vi "BinaryRectangleDetector.vi"(0 "Image In":T2, 7 "error in":errorcluster) -> (20 "Image Out":T2, 21 "distance":dbl, 22 "theta":dbl, 23 "deltax":dbl, 24 "deltay":dbl, 27 "error out":errorcluster)   [LabVIEW 2011]
uses:
  <vilib>/vision/Image Controls.llb/IMAQ Image.ctl
  <vilib>/vision/Measure.llb/Edge Options.ctl
  <vilib>/vision/Measure.llb/Edge Polarity.ctl
  <vilib>/vision/Measure.llb/Straight Edge Options.ctl
  <vilib>/vision/Measure.llb/Straight Edge Process.ctl
  <vilib>/vision/NI_Vision_Development_Module.lvlib
  <vilib>/Analysis/NI_AALBase.lvlib
panel:
  in  "Use Simple":bool
  out "Simple Height":dbl
  out "Simple Width":dbl
  in  "db":dbl=3.0
  in  "thresh":dbl=300.0
  out "width":sgl
  out "height":sgl
  in  "d0":dbl=115.0
  in  "p0":dbl=63.0
  in  "Rectangle":T1 {"Rotation" format="%.2f"; "Left" scale=0.0..1024.0; "Right" scale=0.0..1024.0}
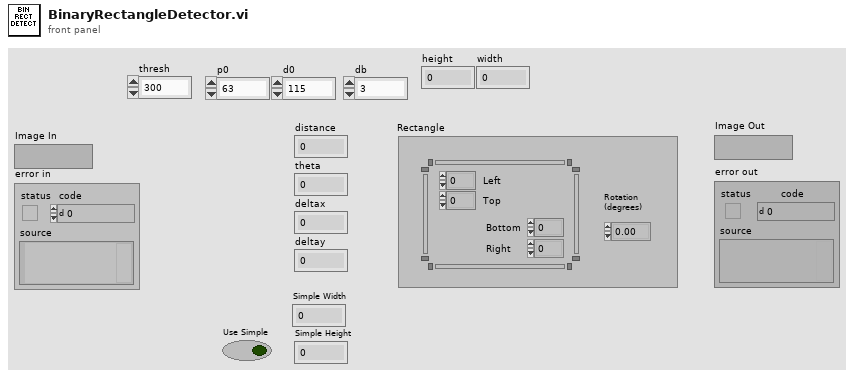
[diagram p1: front panel]
types:
  T1 = typedef "IMAQ Rectangle" = cluster{"Left":i32, "Top":i32, "Right":i32, "Bottom":i32, "Rotation":dbl}
  T2 = typedef "IMAQ Image.ctl" = refnum<image>
  T3 = cluster{"Feature":u32, "Points IDs":cluster{"GUID":string, "Index":i32}[]}[]
  T4 = typedef "Edge Options.ctl" = cluster{"Edge Polarity":T5, "Kernel Size":u32, "Width":u32, "Minimum Edge Strength":sgl, "Interpolation Type":enum32{"Zero Order", "Bilinear", "Quadratic", "Cubic", "Bilinear Fixed"}, "Data Processing Method":enum32{"Average", "Median"}}
  T5 = typedef "Edge Polarity.ctl" = u32
  T6 = cluster{"Search Direction":u32, "Edge Options":T4, "Show Search Area":bool, "Show Search Lines":bool, "Show Edges Found":bool, "Show Result":bool, "Search Area Color":u32, "Search Lines Color":u32, "Edge Locations Color":u32, "Result Color":u32, "Overlay Group Name":string}
  T7 = typedef "Straight Edge Options.ctl" = cluster{"Number of Lines":i32, "Type":T8, "Min. Score":dbl, "Max. Score":dbl, "Orientation":dbl, "Angle Range":dbl, "Angle Tolerance":dbl, "Step Size":u32, "Min. SNR (db)":dbl, "Min. Points (%)":dbl, "Hough Iterations":i32}
  T8 = typedef "Straight Edge Process.ctl" = enum32{"First Edge Rake", "Best Edge Rake", "Hough Edge Rake", "First Edge Projection", "Best Edge Projection"}
  T9 = typedef "ROI Descriptor" = cluster{"Global Rectangle":i32[], "Contours":cluster{"ID":enum32{"External", "Internal"}, "Type":u32, "Coordinates":i32[]}[]}
  T10 = cluster{"histogram":u32[], "Minimal Value":sgl, "Maximal Value":sgl, "Starting Value":sgl, "Interval Width":sgl, "Mean Value":sgl, "Standard  Variation":sgl, "Area (pixels)":i32}
  T11 = typedef "Image Type" = u32
  T12 = cluster{"Point1 (Pixels)":cluster{"X":sgl, "Y":sgl}, "Point2 (Pixels)":cluster{"X":sgl, "Y":sgl}, "Point1 (Real-World)":cluster{"X":sgl, "Y":sgl}, "Point2 (Real-World)":cluster{"X":sgl, "Y":sgl}, "Angle (Pixel)":dbl, "Angle (Real-World)":dbl, "Score":dbl, "Straightness":dbl, "Average SNR (db)":dbl, "Calibration Valid":bool}[]
  T13 = cluster{"Point1 (Pixels)":cluster{"X":sgl, "Y":sgl}, "Point2 (Pixels)":cluster{"X":sgl, "Y":sgl}, "Point1 (Real-World)":cluster{"X":sgl, "Y":sgl}, "Point2 (Real-World)":cluster{"X":sgl, "Y":sgl}, "Angle (Pixel)":dbl, "Angle (Real-World)":dbl, "Score":dbl, "Straightness":dbl, "Average SNR (db)":dbl, "Calibration Valid":bool}
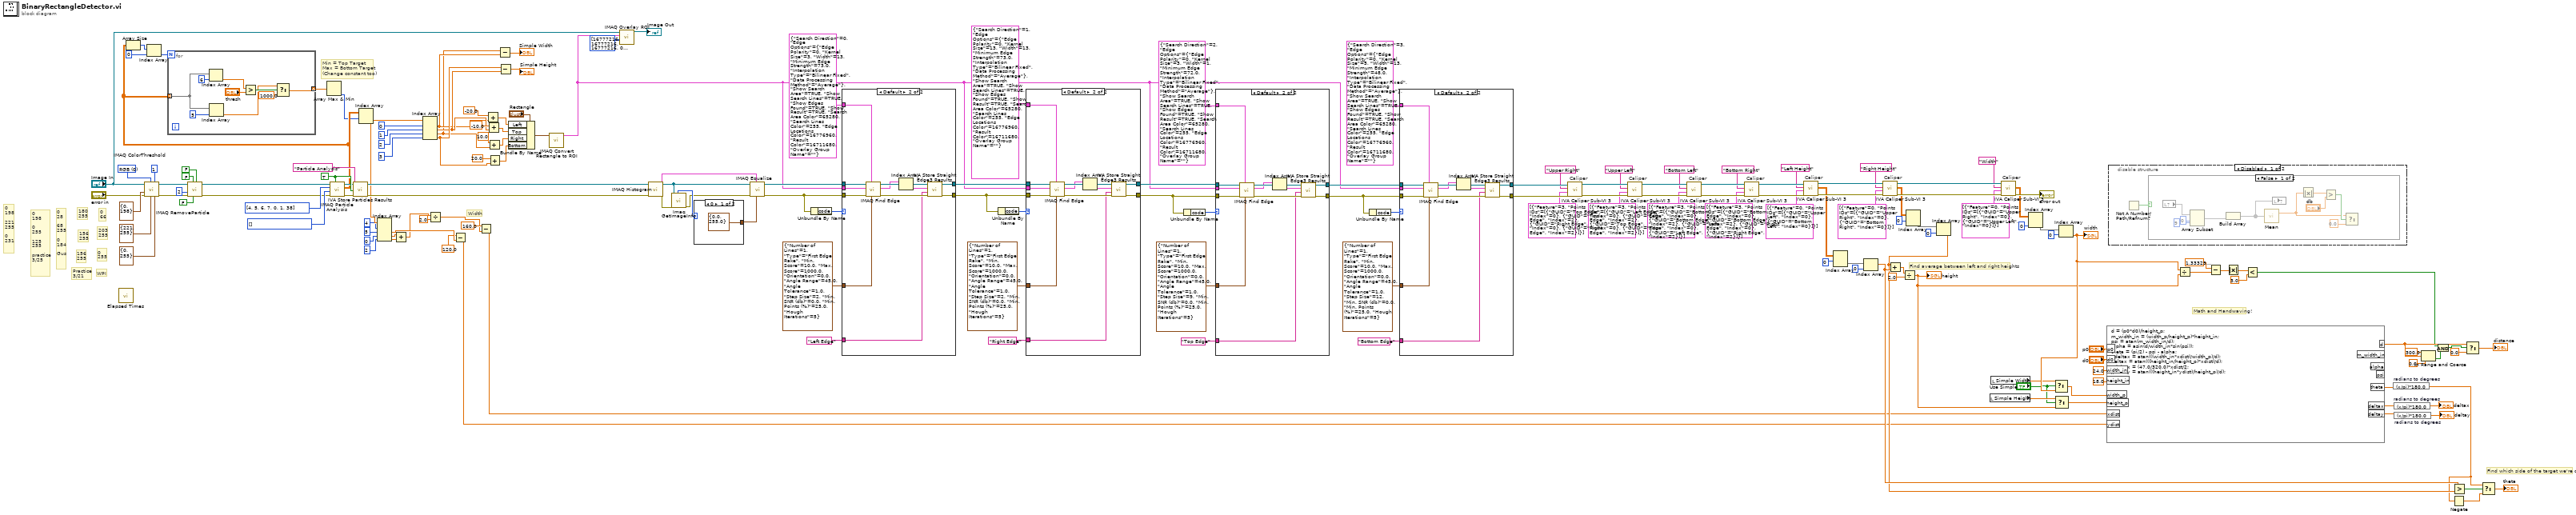
[diagram p0: block diagram]
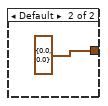
[diagram p8: hidden frame]
diagram:
  w162 = i32[] [] items=["Center of Mass X", "Center of Mass Y", "First Pixel X", "First Pixel Y", "Bounding Rect Left", "Bounding Rect Top", "Bounding Rect Right", "Bounding Rect Bottom", "Max Feret Diameter Start X", "Max Feret Diameter Start Y", "Max Feret Diameter End X", "Max Feret Diameter End Y", "Max Horiz. Segment Length Left", "Max Horiz. Segment Length Right", "Max Horiz. Segment Length Row", "-", "Bounding Rect Width", "Bounding Rect Height", "Bounding Rect Diagonal", "Perimeter", "Convex Hull Perimeter", "Holes' Perimeter", "Max Feret Diameter", "Equivalent Ellipse Major Axis", "Equivalent Ellipse Minor Axis", "Equivalent Ellipse Minor Axis (Feret)", "Equivalent Rect Long Side", "Equivalent Rect Short Side", "Equivalent Rect Diagonal", "Equivalent Rect Short Side (Feret)", "Average Horiz. Segment Length", "Average Vert. Segment Length", "Hydraulic Radius", "Waddel Disk Diameter", "-", "Area", "Holes' Area", "Particle & Holes' Area", "Convex Hull Area", "Image Area", "-", "Number of Holes", "Number of Horiz. Segments", "Number of Vert. Segments", "-", "Orientation", "Max Feret Diameter Orientation", "-", "% Area/Image Area", "% Area/(Particle & Holes' Area)", "Ratio of Equivalent Ellipse Axes", "Ratio of Equivalent Rect Sides", "-", "Elongation Factor", "Compactness Factor", "Heywood Circularity Factor", "Type Factor", "-", "Sum X", "Sum Y", "Sum XX", "Sum XY", "Sum YY", "Sum XXX", "Sum XXY", "Sum XYY", "Sum YYY", "-", "Moment of Inertia XX", "Moment of Inertia XY", "Moment of Inertia YY", "Moment of Inertia XXX", "Moment of Inertia XXY", "Moment of Inertia XYY", "Moment of Inertia YYY", "Norm. Moment of Inertia XX", "Norm. Moment of Inertia XY", "Norm. Moment of Inertia YY", "Norm. Moment of Inertia XXX", "Norm. Moment of Inertia XXY", "Norm. Moment of Inertia XYY", "Norm. Moment of Inertia YYY", "Hu Moment 1", "Hu Moment 2", "Hu Moment 3", "Hu Moment 4", "Hu Moment 5", "Hu Moment 6", "Hu Moment 7"] ("Real-World Measurements")
  w163 = i32[] [4, 5, 6, 7, 0, 1, 38] items=["Center of Mass X", "Center of Mass Y", "First Pixel X", "First Pixel Y", "Bounding Rect Left", "Bounding Rect Top", "Bounding Rect Right", "Bounding Rect Bottom", "Max Feret Diameter Start X", "Max Feret Diameter Start Y", "Max Feret Diameter End X", "Max Feret Diameter End Y", "Max Horiz. Segment Length Left", "Max Horiz. Segment Length Right", "Max Horiz. Segment Length Row", "-", "Bounding Rect Width", "Bounding Rect Height", "Bounding Rect Diagonal", "Perimeter", "Convex Hull Perimeter", "Holes' Perimeter", "Max Feret Diameter", "Equivalent Ellipse Major Axis", "Equivalent Ellipse Minor Axis", "Equivalent Ellipse Minor Axis (Feret)", "Equivalent Rect Long Side", "Equivalent Rect Short Side", "Equivalent Rect Diagonal", "Equivalent Rect Short Side (Feret)", "Average Horiz. Segment Length", "Average Vert. Segment Length", "Hydraulic Radius", "Waddel Disk Diameter", "-", "Area", "Holes' Area", "Particle & Holes' Area", "Convex Hull Area", "Image Area", "-", "Number of Holes", "Number of Horiz. Segments", "Number of Vert. Segments", "-", "Orientation", "Max Feret Diameter Orientation", "-", "% Area/Image Area", "% Area/(Particle & Holes' Area)", "Ratio of Equivalent Ellipse Axes", "Ratio of Equivalent Rect Sides", "-", "Elongation Factor", "Compactness Factor", "Heywood Circularity Factor", "Type Factor", "-", "Sum X", "Sum Y", "Sum XX", "Sum XY", "Sum YY", "Sum XXX", "Sum XXY", "Sum XYY", "Sum YYY", "-", "Moment of Inertia XX", "Moment of Inertia XY", "Moment of Inertia YY", "Moment of Inertia XXX", "Moment of Inertia XXY", "Moment of Inertia XYY", "Moment of Inertia YYY", "Norm. Moment of Inertia XX", "Norm. Moment of Inertia XY", "Norm. Moment of Inertia YY", "Norm. Moment of Inertia XXX", "Norm. Moment of Inertia XXY", "Norm. Moment of Inertia XYY", "Norm. Moment of Inertia YYY", "Hu Moment 1", "Hu Moment 2", "Hu Moment 3", "Hu Moment 4", "Hu Moment 5", "Hu Moment 6", "Hu Moment 7"] ("Pixel Measurements")
  w161 = TRUE ("Connectivity 4/8 (8)")
  w173 = u16 0 items=["RGB", "HSL", "HSV", "HSI"] ("Color Mode")
  # "Width"
  # "0\n198\n\n221\n255\n\n0\n231"
  # "0\n198\n\n0\n255\n\n125\n255\n\npractice\n3/25"
  # "0\n28\n\n68\n255\n\n0\n184\n\nGus"
  # "Practice\n3/21"
  # "WPI"
  # "156\n255"
  # "156\n255"
  # "180\n255"
  # "0\n255"
  # "203\n255"
  # "0\n66"
  # "Min = Top Target\nMax = Bottom Target\n(Change constant too)"
  # "Find average between left and right heights"
  # "Math and Handwaving!"
  # "Find which side of the target we're on"
  # "Caliper"
  # "Caliper"
  # "Caliper"
  # "Caliper"
  # "Caliper"
  # "Caliper"
  # "Caliper"
  n1 = call "Elapsed Times.vi"() -> ()  [unwired: 3 in, 1 out]
  n2 = call "IMAQ ColorThreshold"("Blue or Luma or Val or Inten Range"=cluster{"Lower value":i32, "Upper value":i32} {"Lower value"=0, "Upper value"=255}, "Replace Value"=1, "Green or Sat Range"=cluster{"Lower value":i32, "Upper value":i32} {"Lower value"=221, "Upper value"=255}, "Color Mode"=w173, "error in (no error)"="error in", "Red or Hue Range"=cluster{"Lower value":i32, "Upper value":i32} {"Lower value"=0, "Upper value"=198}, "Image Src"="Image In") -> ("error out"=w168:errorcluster, "Image Dst Out"=w39:T2)  [unwired: 1 in, 2 out]
  n3 = call "IMAQ RemoveParticle"("Connectivity 4/8 (8)"=FALSE, "Low Pass/High Pass (Low)"=FALSE, "Square/Hexa (Square)"=FALSE, "error in (no error)"=w168, "Number of Erosion"=2, "Image Src"=w39) -> ("error out"=w41:errorcluster, "Image Dst Out"=w42:T2)  [unwired: 1 in, 3 out]
  n4 = call "IMAQ Particle Analysis"("Connectivity 4/8 (8)"=w161, "error in (no error)"=w41, "Real-World Measurements"=w162, "Pixel Measurements"=w163, "Image"=w42) -> ("error out"=w158:errorcluster, "Particle Measurements (Pixels)"=w36:dbl[][], "Image Out (duplicate)"=w160:T2)  [unwired: 4 out]
  n5 = Array Size(array=w36) -> (size(s)=w50:i32[])
  n6 = Index Array(array=w50, index=0) -> (element=w48:i32)
  n7 = for {
    N: w48 -> [_]
    tunnel: w36 -> [w181] mode=indexing
    tunnel: [w175] -> w40 mode=indexing
    n8 = Index Array(array=w181, index=6) -> (element=w180:dbl)
    n9 = Index Array(array=w181, index=5) -> (element=w177:dbl)
    n10 = Greater?(x=w180, y="thresh") -> (0:w178:bool)
    n11 = Select(t=w177, s=w178, f=1000.0) -> (s? t:f=w175:dbl)
  }
  n12 = Array Max & Min(array=w40) -> (min index (indices)=w29:i32)  [unwired: 3 out]
  n13 = call <vilib>:"IVA Store Particles Results.vi"("error in (no error)"=w158, "Connectivity 4/8 (8)"=w161, "Step Name"="Particle Analysis", "Image in"=w160) -> ("error out"=w157:errorcluster, "Image dup"=w153:T2)  [unwired: 6 out]
  n14 = Index Array(array=w36, index (row)=w29) -> (element=w69:dbl[])  [unwired: 1 in]
  n15 = Index Array(array=w69, index #1=4 ("index"), index #2=5 ("index"), index #3=0 ("index"), index #4=2 ("index")) -> (element #2=w45:dbl, element #3=w5:dbl, element #4=w4:dbl)  [unwired: 1 out]
  n16 = Add(x=w5, y=w4) -> (x+y=w3:dbl)
  n17 = Index Array(array=w69, index #1=0 ("index"), index #2=1 ("index"), index #3=2 ("index"), index #4=3 ("index")) -> (element #1=w17:dbl, element #2=w18:dbl, element #3=w16:dbl, element #4=w19:dbl)
  n18 = Divide(x=w3, y=2.0) -> (x/y=w1:dbl)
  n19 = Subtract(x=120.0, y=w45) -> (x-y=w43:dbl)
  n20 = Subtract(x=160.0, y=w1) -> (x-y=w46:dbl)
  n21 = Add(x=-20.0 ("y"), y=w17) -> (x+y=w90:dbl)
  n22 = Add(x=-10.0, y=w18) -> (x+y=w89:dbl)
  n23 = Add(x=10.0, y=w16) -> (x+y=w88:dbl)
  n24 = Add(x=20.0, y=w19) -> (x+y=w87:dbl)
  n25 = Subtract(x=w16, y=w17) -> (x-y=→"Simple Width":dbl)
  n26 = Subtract(x=w19, y=w18) -> (x-y=→"Simple Height":dbl)
  n27 = Bundle By Name(cluster="Rectangle", "Left"=w90, "Top"=w89, "Right"=w88, "Bottom"=w87) -> (w86:T1)
  n28 = call "IMAQ Convert Rectangle to ROI"("Rectangle"=w86) -> ("ROI Descriptor"=w37:T9)  [unwired: 8 in, 1 out]
  n29 = call "IMAQ Overlay ROI"("Point Symbol"=u32[][] [[16777216, 16777216, 16777216, 0, 16777216, 16777216, 16777216], [16777216, 16777216, 16777216, 0, 16777216, 16777216, 16777216], [16777216, 16777216, 16777216, 0, 16777216, 16777216, 16777216], [0, 0, 0, 16777216, 0, 0, 0], [16777216, 16777216, 16777216, 0, 16777216, 16777216, 16777216], [16777216, 16777216, 16777216, 0, 16777216, 16777216, 16777216], [16777216, 16777216, 16777216, 0, 16777216, 16777216, 16777216]], "ROI Descriptor"=w37, "Image"="Image In") -> ("Image Out"=→"Image Out":T2)  [unwired: 7 in, 1 out]
  n30 = call "IMAQ Histogram"("error in (no error)"=w157, "Image"=w153) -> ("error out"=w152:errorcluster, "Histogram Report"=w155:T10)  [unwired: 3 in, 5 out]
  n31 = call "Imaq GetImageInfo"("error in (no error)"=w152, "Image"=w153) -> ("error out"=w151:errorcluster, "Image Type"=w154:T11)  [unwired: 8 out]
  n32 = case shown="0" w154 {
    tunnel: [cluster{"Minimum":sgl, "Maximum":sgl} {"Minimum"=0.0, "Maximum"=255.0} ("Range") cluster{"Minimum":sgl, "Maximum":sgl} {"Minimum"=0.0, "Maximum"=0.0} ("Range")] -> w150
    frame 0 {
    }
    frame Default {
    }
  }
  n33 = call "IMAQ Equalize"("Range"=w150, "Histogram Report"=w155, "error in (no error)"=w151, "Image Src"=w153) -> ("error out"=w156:errorcluster, "Image Dst Out"=w85:T2)  [unwired: 2 in, 4 out]
  n34 = Unbundle By Name(w156) -> ("code"=w147:i32)
  n35 = case shown="Default" w147 {
    tunnel: w85 -> [w186 w198]
    tunnel: w156 -> [_ w197]
    tunnel: w37 -> [_ w191]
    tunnel: [w186 w195] -> w144
    tunnel: [_ w193] -> w149
    tunnel: "Left Edge" ("Step Name") -> [_ w192]
    tunnel: T7 {"Number of Lines"=1, "Type"=enum."First Edge Rake", "Min. Score"=10.0, "Max. Score"=1000.0, "Orientation"=0.0, "Angle Range"=45.0, "Angle Tolerance"=1.0, "Step Size"=2, "Min. SNR (db)"=0.0, "Min. Points (%)"=25.0, "Hough Iterations"=5} ("Fit Options") -> [_ w190]
    tunnel: T6 {"Search Direction"=0, "Edge Options"={"Edge Polarity"=0, "Kernel Size"=3, "Width"=13, "Minimum Edge Strength"=73.0, "Interpolation Type"=enum."Bilinear Fixed", "Data Processing Method"=enum."Average"}, "Show Search Area"=TRUE, "Show Search Lines"=TRUE, "Show Edges Found"=TRUE, "Show Result"=TRUE, "Search Area Color"=65280, "Search Lines Color"=255, "Edge Locations Color"=16776960, "Result Color"=16711680, "Overlay Group Name"=""} ("Options") -> [_ w189]
    frame -1074396199, -1074396198 {
      # "Discard Coordinate System Error"
    }
    frame Default {
      n36 = call "IMAQ Find Edge"("Line Fit Options"=w190, "Options"=w189, "error in (no error)"=w197, "ROI Descriptor"=w191, "Image"=w198) -> ("error out"=w194:errorcluster, "Straight Edges"=w188:T12, "Image Out"=w196:T2)  [unwired: 1 in, 3 out]
      n37 = Index Array(array=w188) -> (element=w187:T13)  [unwired: 1 in]
      n38 = call <vilib>:"IVA Store Straight Edge3 Results.vi"("error in (no error)"=w194, "Step Name"=w192, "Straight Edge"=w187, "Image in"=w196) -> ("error out"=w193:errorcluster, "Image dup"=w195:T2)  [unwired: 1 in, 5 out]
    }
  }
  n39 = Unbundle By Name(w149) -> ("code"=w141:i32)
  n40 = case shown="Default" w141 {
    tunnel: w144 -> [w199 w211]
    tunnel: w149 -> [_ w210]
    tunnel: w37 -> [_ w204]
    tunnel: [w199 w208] -> w138
    tunnel: [_ w206] -> w143
    tunnel: "Right Edge" ("Step Name") -> [_ w205]
    tunnel: T7 {"Number of Lines"=1, "Type"=enum."First Edge Rake", "Min. Score"=10.0, "Max. Score"=1000.0, "Orientation"=0.0, "Angle Range"=45.0, "Angle Tolerance"=1.0, "Step Size"=2, "Min. SNR (db)"=0.0, "Min. Points (%)"=25.0, "Hough Iterations"=5} ("Fit Options") -> [_ w203]
    tunnel: T6 {"Search Direction"=1, "Edge Options"={"Edge Polarity"=0, "Kernel Size"=13, "Width"=13, "Minimum Edge Strength"=73.0, "Interpolation Type"=enum."Bilinear Fixed", "Data Processing Method"=enum."Average"}, "Show Search Area"=TRUE, "Show Search Lines"=TRUE, "Show Edges Found"=TRUE, "Show Result"=TRUE, "Search Area Color"=65280, "Search Lines Color"=255, "Edge Locations Color"=16776960, "Result Color"=16711680, "Overlay Group Name"=""} ("Options") -> [_ w202]
    frame -1074396199, -1074396198 {
      # "Discard Coordinate System Error"
    }
    frame Default {
      n41 = call "IMAQ Find Edge"("Line Fit Options"=w203, "Options"=w202, "error in (no error)"=w210, "ROI Descriptor"=w204, "Image"=w211) -> ("error out"=w207:errorcluster, "Straight Edges"=w201:T12, "Image Out"=w209:T2)  [unwired: 1 in, 3 out]
      n42 = Index Array(array=w201) -> (element=w200:T13)  [unwired: 1 in]
      n43 = call <vilib>:"IVA Store Straight Edge3 Results.vi"("error in (no error)"=w207, "Step Name"=w205, "Straight Edge"=w200, "Image in"=w209) -> ("error out"=w206:errorcluster, "Image dup"=w208:T2)  [unwired: 1 in, 5 out]
    }
  }
  n44 = Unbundle By Name(w143) -> ("code"=w135:i32)
  n45 = case shown="Default" w135 {
    tunnel: w138 -> [w212 w224]
    tunnel: w143 -> [_ w223]
    tunnel: [w212 w221] -> w132
    tunnel: [_ w219] -> w137
    tunnel: "Top Edge" ("Step Name") -> [_ w218]
    tunnel: T7 {"Number of Lines"=1, "Type"=enum."First Edge Rake", "Min. Score"=10.0, "Max. Score"=1000.0, "Orientation"=0.0, "Angle Range"=45.0, "Angle Tolerance"=1.0, "Step Size"=9, "Min. SNR (db)"=0.0, "Min. Points (%)"=25.0, "Hough Iterations"=5} ("Fit Options") -> [_ w217]
    tunnel: T6 {"Search Direction"=2, "Edge Options"={"Edge Polarity"=0, "Kernel Size"=3, "Width"=1, "Minimum Edge Strength"=72.0, "Interpolation Type"=enum."Bilinear Fixed", "Data Processing Method"=enum."Average"}, "Show Search Area"=TRUE, "Show Search Lines"=TRUE, "Show Edges Found"=TRUE, "Show Result"=TRUE, "Search Area Color"=65280, "Search Lines Color"=255, "Edge Locations Color"=16776960, "Result Color"=16711680, "Overlay Group Name"=""} ("Options") -> [_ w216]
    tunnel: w37 -> [_ w213]
    frame -1074396199, -1074396198 {
      # "Discard Coordinate System Error"
    }
    frame Default {
      n46 = call "IMAQ Find Edge"("Line Fit Options"=w217, "Options"=w216, "error in (no error)"=w223, "ROI Descriptor"=w213, "Image"=w224) -> ("error out"=w220:errorcluster, "Straight Edges"=w215:T12, "Image Out"=w222:T2)  [unwired: 1 in, 3 out]
      n47 = Index Array(array=w215) -> (element=w214:T13)  [unwired: 1 in]
      n48 = call <vilib>:"IVA Store Straight Edge3 Results.vi"("error in (no error)"=w220, "Step Name"=w218, "Straight Edge"=w214, "Image in"=w222) -> ("error out"=w219:errorcluster, "Image dup"=w221:T2)  [unwired: 1 in, 5 out]
    }
  }
  n49 = Unbundle By Name(w137) -> ("code"=w129:i32)
  n50 = case shown="Default" w129 {
    tunnel: w132 -> [w225 w237]
    tunnel: w137 -> [_ w236]
    tunnel: w37 -> [_ w230]
    tunnel: [w225 w234] -> w126
    tunnel: [_ w232] -> w131
    tunnel: "Bottom Edge" ("Step Name") -> [_ w231]
    tunnel: T7 {"Number of Lines"=1, "Type"=enum."First Edge Rake", "Min. Score"=10.0, "Max. Score"=1000.0, "Orientation"=0.0, "Angle Range"=45.0, "Angle Tolerance"=1.0, "Step Size"=12, "Min. SNR (db)"=0.0, "Min. Points (%)"=25.0, "Hough Iterations"=5} ("Fit Options") -> [_ w229]
    tunnel: T6 {"Search Direction"=3, "Edge Options"={"Edge Polarity"=0, "Kernel Size"=5, "Width"=13, "Minimum Edge Strength"=48.0, "Interpolation Type"=enum."Bilinear Fixed", "Data Processing Method"=enum."Average"}, "Show Search Area"=TRUE, "Show Search Lines"=TRUE, "Show Edges Found"=TRUE, "Show Result"=TRUE, "Search Area Color"=65280, "Search Lines Color"=255, "Edge Locations Color"=16776960, "Result Color"=16711680, "Overlay Group Name"=""} ("Options") -> [_ w228]
    frame -1074396199, -1074396198 {
      # "Discard Coordinate System Error"
    }
    frame Default {
      n51 = call "IMAQ Find Edge"("Line Fit Options"=w229, "Options"=w228, "error in (no error)"=w236, "ROI Descriptor"=w230, "Image"=w237) -> ("error out"=w233:errorcluster, "Straight Edges"=w227:T12, "Image Out"=w235:T2)  [unwired: 1 in, 3 out]
      n52 = Index Array(array=w227) -> (element=w226:T13)  [unwired: 1 in]
      n53 = call <vilib>:"IVA Store Straight Edge3 Results.vi"("error in (no error)"=w233, "Step Name"=w231, "Straight Edge"=w226, "Image in"=w235) -> ("error out"=w232:errorcluster, "Image dup"=w234:T2)  [unwired: 1 in, 5 out]
    }
  }
  n54 = call <vilib>:"IVA Caliper Sub-VI 3.vi"("error in"=w131, "Parameters"=T3 [{"Feature"=3, "Points IDs"=[{"GUID"="Top Edge", "Index"=0}, {"GUID"="Top Edge", "Index"=2}, {"GUID"="Right Edge", "Index"=0}, {"GUID"="Right Edge", "Index"=2}]}], "Step Name"="Upper Right", "Image In"=w126) -> ("error out"=w125:errorcluster, "Image Out"=w122:T2)  [unwired: 1 in, 5 out]
  n55 = call <vilib>:"IVA Caliper Sub-VI 3.vi"("error in"=w125, "Parameters"=T3 [{"Feature"=3, "Points IDs"=[{"GUID"="Left Edge", "Index"=0}, {"GUID"="Left Edge", "Index"=2}, {"GUID"="Top Edge", "Index"=0}, {"GUID"="Top Edge", "Index"=2}]}], "Step Name"="Upper Left", "Image In"=w122) -> ("error out"=w121:errorcluster, "Image Out"=w118:T2)  [unwired: 1 in, 5 out]
  n56 = call <vilib>:"IVA Caliper Sub-VI 3.vi"("error in"=w121, "Parameters"=T3 [{"Feature"=3, "Points IDs"=[{"GUID"="Bottom Edge", "Index"=0}, {"GUID"="Bottom Edge", "Index"=2}, {"GUID"="Left Edge", "Index"=0}, {"GUID"="Left Edge", "Index"=2}]}], "Step Name"="Bottom Left", "Image In"=w118) -> ("error out"=w117:errorcluster, "Image Out"=w114:T2)  [unwired: 1 in, 5 out]
  n57 = call <vilib>:"IVA Caliper Sub-VI 3.vi"("error in"=w117, "Parameters"=T3 [{"Feature"=3, "Points IDs"=[{"GUID"="Bottom Edge", "Index"=0}, {"GUID"="Bottom Edge", "Index"=2}, {"GUID"="Right Edge", "Index"=0}, {"GUID"="Right Edge", "Index"=2}]}], "Step Name"="Bottom Right", "Image In"=w114) -> ("error out"=w113:errorcluster, "Image Out"=w110:T2)  [unwired: 1 in, 5 out]
  n58 = call <vilib>:"IVA Caliper Sub-VI 3.vi"("error in"=w113, "Parameters"=T3 [{"Feature"=0, "Points IDs"=[{"GUID"="Upper Left", "Index"=0}, {"GUID"="Bottom Left", "Index"=0}]}], "Step Name"="Left Height", "Image In"=w110) -> ("error out"=w109:errorcluster, "Results (Pixels)"=w81:sgl[][], "Image Out"=w106:T2)  [unwired: 1 in, 4 out]
  n59 = Index Array(array=w81, index (row)=0) -> (element=w79:sgl[])  [unwired: 1 in]
  n60 = Index Array(array=w79, index=0) -> (element=w60:sgl)
  n61 = call <vilib>:"IVA Caliper Sub-VI 3.vi"("error in"=w109, "Parameters"=T3 [{"Feature"=0, "Points IDs"=[{"GUID"="Upper Right", "Index"=0}, {"GUID"="Bottom Right", "Index"=0}]}], "Step Name"="Right Height", "Image In"=w106) -> ("error out"=w105:errorcluster, "Results (Pixels)"=w77:sgl[][], "Image Out"=w102:T2)  [unwired: 1 in, 4 out]
  n62 = Index Array(array=w77, index (row)=0) -> (element=w75:sgl[])  [unwired: 1 in]
  n63 = Index Array(array=w75, index=0) -> (element=w59:sgl)
  n64 = Add(x=w59, y=w60) -> (x+y=w62:sgl)
  n65 = Divide(x=w62, y=sgl 2.0) -> (x/y=w22:sgl)
  "height" <- w22
  n66 = local read "Simple Height"() -> (w21:dbl)
  n67 = local read "Simple Width"() -> (w25:dbl)
  n68 = call <vilib>:"IVA Caliper Sub-VI 3.vi"("error in"=w105, "Parameters"=T3 [{"Feature"=0, "Points IDs"=[{"GUID"="Upper Right", "Index"=0}, {"GUID"="Upper Left", "Index"=0}]}], "Step Name"="Width", "Image In"=w102) -> ("error out"=→"error out":errorcluster, "Results (Pixels)"=w73:sgl[][])  [unwired: 1 in, 5 out]
  n69 = Index Array(array=w73, index (row)=0) -> (element=w71:sgl[])  [unwired: 1 in]
  n70 = Select(t=w21, s="Use Simple", f=w22) -> (s? t:f=w23:dbl)
  n71 = Index Array(array=w71, index=0) -> (element=w26:sgl)
  "width" <- w26
  n72 = Select(t=w25, s="Use Simple", f=w26) -> (s? t:f=w24:dbl)
  n73 = formula code="d = (p0*d0)/height_p;\nm_width_in = (width_p/height_p)*height_in;\npsi = atan(m_width_in/d);\nalpha = asin(d/width_in*sin(psi));\ntheta = (pi/2) - psi - alpha;\n//deltax = atan(((width_in*xdist)/width_p)/d);\ndeltax = atan(((height_in/height_p)*xdist)/d);\n//deltax = (47.0/320.0)*xdist/2;\n//deltay = atan(((height_in*ydist)/height_p)/d);"("p0"="p0", "d0"="d0", "width_in"=24.0 ("input variable"), "height_in"=18.0 ("input variable"), "height_p"=w23, "width_p"=w24, "xdist"=w46, "ydist"=w43) -> ("d"=w13:dbl, "theta"=w57:dbl, "deltax"=w54:dbl, "deltay"=w53:dbl)  [unwired: 3 out]
  n74 = disable-structure shown="Disabled" {
    frame Disabled {
      n75 = Not A Number/Path/Refnum?() -> (NaN/Path/Refnum?=w238:bool)  [unwired: 1 in]
      n76 = case shown="False" w238 {
        frame False {
          n77 = local read item#-1() -> (w248)
          n78 = Array Subset(array=w248, index=0, length=9) -> (w246:void[])
          n79 = Build Array(w246) -> (w245:void[])  [unwired: 1 in]
          n80 = call <vilib>:"Mean.vi"("X"=w245) -> ("mean"=w239:dbl)  [unwired: 1 out]
          n81 = local write item#-1(w245) -> ()
          n82 = Absolute Value(x=w239) -> (abs(x)=w241:dbl)
          n83 = Greater?(x=w241, y="db") -> (0:w243:bool)
          n84 = Select(t=w239, s=w243, f=0.0) -> ()  [unwired: 1 out]
        }
        frame True {
        }
      }
    }
    frame Enabled {
    }
  }
  n85 = Divide(x=w26, y=w22) -> (x/y=w35:sgl)
  n86 = Subtract(x=sgl 1.3333, y=w35) -> (x-y=w33:sgl)
  n87 = Absolute Value(x=w33) -> (abs(x)=w32:sgl)
  n88 = Less?(x=w32, y=sgl 3.0) -> (x < y?=w8:bool)
  n89 = expression code="(x/pi)*180.0" "radians to degrees"(w57) -> (w55:dbl)
  n90 = expression code="(x/pi)*180.0" "radians to degrees"(w54) -> (→"deltax":dbl)
  n91 = expression code="(x/pi)*180.0" "radians to degrees"(w53) -> (→"deltay":dbl)
  n92 = In Range and Coerce(upper limit=300.0, x=w13, lower limit=0.0) -> (In Range?=w9:bool)  [unwired: 1 out]
  n93 = And(x=w8, y=w9) -> (x .and. y?=w10:bool)
  n94 = Negate(x=w55) -> (-x=w56:dbl)
  n95 = Greater?(x=w60, y=w59) -> (0:w58:bool)
  n96 = Select(t=w13, s=w10, f=0.0) -> (s? t:f=→"distance":dbl)
  n97 = Select(t=w55, s=w58, f=w56) -> (s? t:f=→"theta":dbl)
